vi "Actor Core.vi"(8 "error in":errorcluster, 11 "PLCMonitor in":refnum<class "PLCMonitor.lvclass">) -> (0 "error out":errorcluster, 3 "Actor out":refnum<class "Actor.lvclass">)   [LabVIEW 2020, in "PLCMonitor.lvlib" / "PLCMonitor.lvclass"]
doc: "(<B>Filename</B>: Actor Framework.lvlib:Actor.lvclass:Actor Core.vi)\n\nReceives messages to the actor, reacts to them, and initiates any error handling that may shut the actor down.\n\nDescendant classes may override this VI to append parallel tasks for the actor to complete while it handles messages. Overrides use the Call Parent Class Method node."
uses:
  PLCMonitor.lvclass
  C:/Program Files/National Instruments/LabVIEW 2020/vi.lib/ActorFramework/Actor/Actor.lvclass
  <vilib>/ActorFramework/Actor/Actor.lvclass
  <vilib>/ActorFramework/Actor/Actor.lvclass/Actor.ctl
  <vilib>/ActorFramework/Message Enqueuer/Message Enqueuer.lvclass/Message Enqueuer.ctl
  <vilib>/ActorFramework/Message Enqueuer/Init from Existing Queue.vi
  <vilib>/gpm_packages/@cs/mva-core/Source/IModel/IModel/IModel.lvclass
  <vilib>/ActorFramework/Message Enqueuer/Message Enqueuer.lvclass
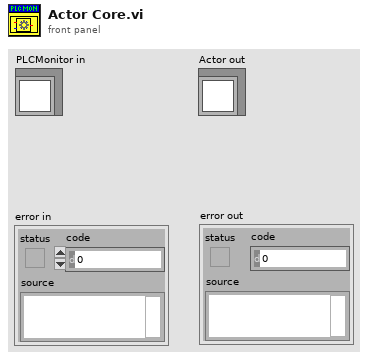
[diagram p1: front panel]
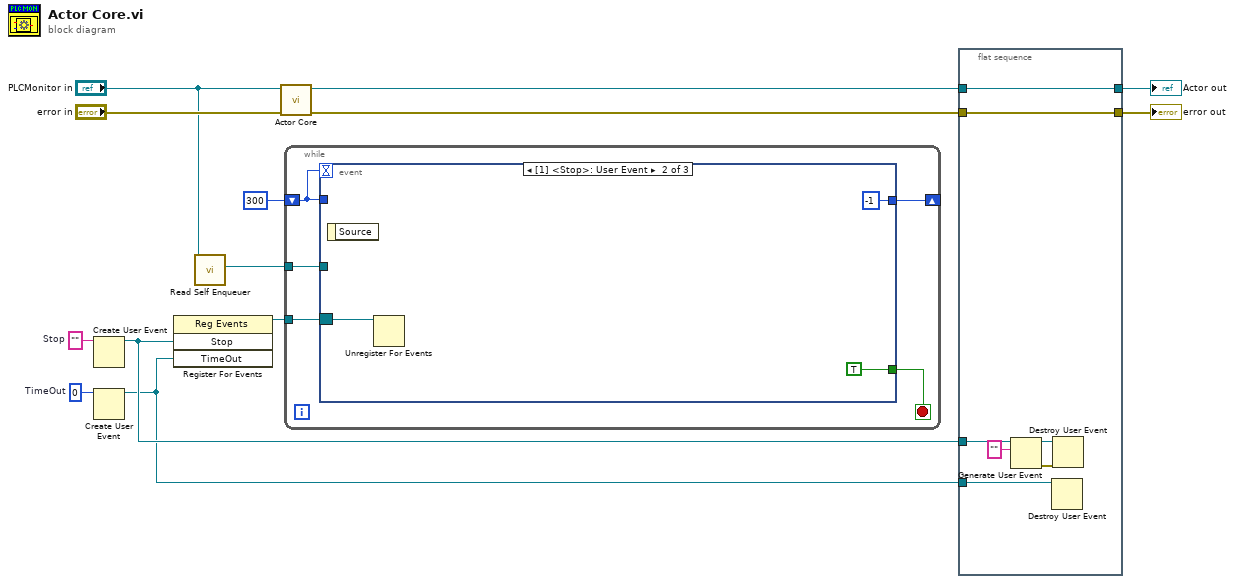
[diagram p0: block diagram]
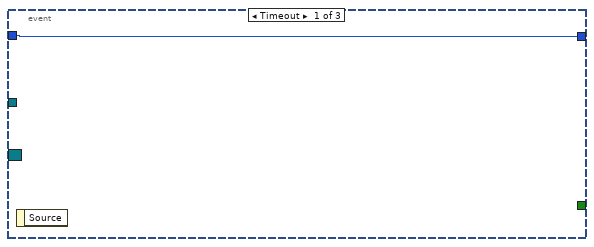
[diagram p2: hidden frame]
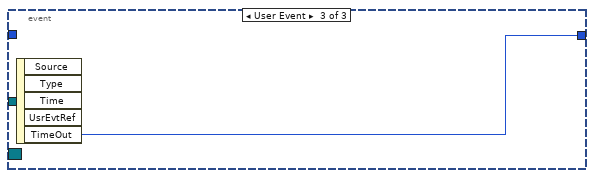
[diagram p3: hidden frame]
diagram:
  w10 = 0  # TimeOut
  w12 = ""  # Stop
  n1 = Create User Event(user event datatype=w12) -> (user event=w7:refnum<user-event>)  [unwired: 1 in, 1 out]
  n2 = Create User Event(user event datatype=w10) -> (user event=w6:refnum<user-event>)  [unwired: 1 in, 1 out]
  n3 = register-events(w7, w6) -> (reference out=w11:refnum<event-registration>)  [unwired: 2 in, 1 out]
  n4 = call <vilib>:"Read Self Enqueuer.vi"("Actor"="PLCMonitor in") -> ("Self Enqueuer"=w1:refnum<class "Message Enqueuer.lvclass">)  [unwired: 10 in]
  n5 = call-parent "Actor Core.vi"("error in"="error in", "Actor in"="PLCMonitor in") -> ("error out"=w4:errorcluster, "Actor out"=w8:refnum<class "Actor.lvclass">)  [unwired: 8 in]
  n6 = while {
    tunnel: w11 -> [w18]
    shift-right: [w16] -> _
    shift-left: 300 -> [w17]
    tunnel: w1 -> [w14]
    stop <- w15 stop-if-true
    n7 = event shown="[1] <Stop>: User Event" {
      selector: w18 -> [_ w21 _]
      dyn-events: _ -> [_ _ _]
      timeout: w17 -> [_ _ _]
      tunnel: w17 -> [w19 _ _]
      tunnel: [w19 -1 ("TimeOut") w23] -> w16
      tunnel: [_ TRUE _] -> w15
      tunnel: w14 -> [_ _ _]
      event Timeout {
        n8 = event-data() -> ()  [unwired: 1 in, 1 out]
      }
      event User Event {
        n9 = event-data() -> ()  [unwired: 1 in, 1 out]
        n10 = Unregister For Events(event registration refnum=w21) -> ()  [unwired: 1 in, 1 out]
      }
      event User Event {
        n11 = event-data() -> ("TimeOut"=w23:i32)  [unwired: 1 in, 4 out]
      }
    }
  }
  n12 = flat-sequence {
    tunnel: [w27] -> w9
    tunnel: w8 -> [w27]
    tunnel: w7 -> [w26]
    tunnel: w6 -> [w25]
    tunnel: [w24] -> w5
    tunnel: w4 -> [w24]
    frame #0 {
      n13 = Generate User Event(user event=w26, event data cluster="" ("event data")) -> (user event out=w30:refnum<user-event>, error out=w29:errorcluster)  [unwired: 2 in]
      n14 = Destroy User Event(user event=w25) -> ()  [unwired: 1 in, 1 out]
      n15 = Destroy User Event(user event=w30, error in=w29) -> ()  [unwired: 1 out]
    }
  }
  "error out" <- w5
  "Actor out" <- w9
